vi "Test Process Restarting Maintains State.vi"(8 "error in (no error)":errorcluster, 11 "Process Test In":refnum<class "Process Test.lvclass">) -> (0 "error out":errorcluster, 3 "Process Test Out":refnum<class "Process Test.lvclass">)   [LabVIEW 2020, in "Process Test.lvclass"]
uses:
  Process Test.lvclass
  <vilib>/Asteme/LUnit/Test Case.lvclass
  C:/Program Files (x86)/National Instruments/LabVIEW 2020/vi.lib/Asteme/LUnit/Test Case.lvclass
  Framework/Process/Process.lvclass
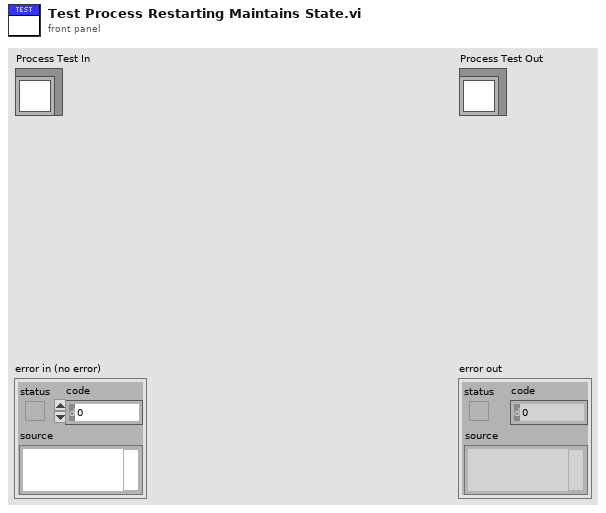
[diagram p1: front panel]
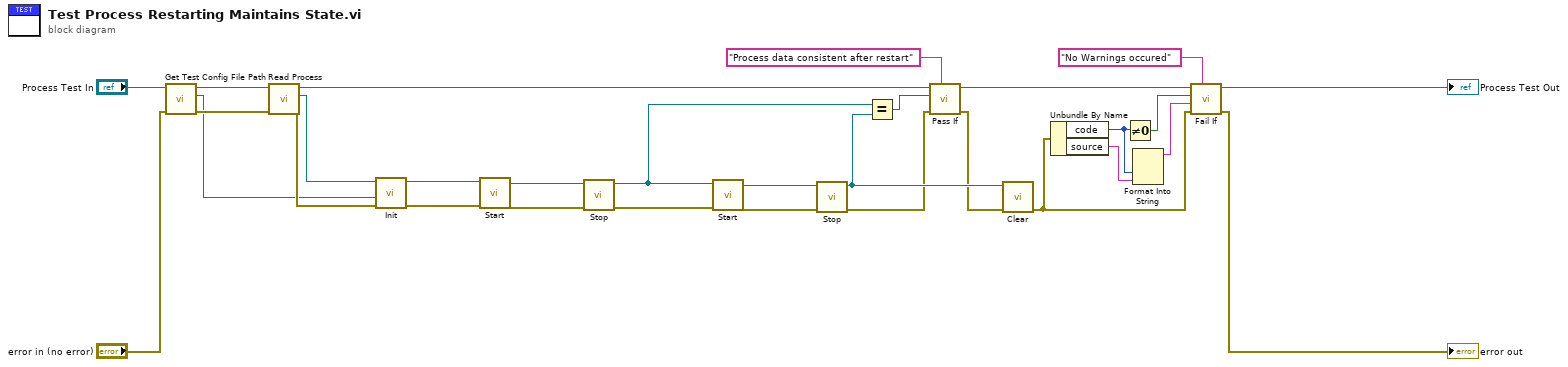
[diagram p0: block diagram]
diagram:
  n1 = call-dynamic "Get Test Config File Path.vi"("error in (no error)"="error in (no error)", "Base Class Test in"="Process Test In") -> ("error out"=w21:errorcluster, "Test config path"=w1:path, "Base Class Test out"=w25:refnum<class "Process Test.lvclass">)  [unwired: 7 in]
  n2 = call "Read Process.vi"("error in (no error)"=w21, "Process Test in"=w25) -> ("error out"=w22:errorcluster, "Process.lvclass"=w2:refnum<class "Process.lvclass">, "Process Test out"=w23:refnum<class "Process Test.lvclass">)  [unwired: 7 in]
  n3 = call-dynamic "Init.vi"("error in (no error)"=w22, "Config File Path"=w1, "Process In"=w2) -> ("error out"=w26:errorcluster, "Process Out"=w27:refnum<class "Process.lvclass">)  [unwired: 7 in]
  n4 = call "Start.vi"("error in (no error)"=w26, "Process In"=w27) -> ("error out"=w29:errorcluster, "Process Out"=w30:refnum<class "Process.lvclass">)  [unwired: 8 in]
  n5 = call "Stop.vi"("error in (no error)"=w29, "Process In"=w30) -> ("error out"=w3:errorcluster, "Process Out"=w10:refnum<class "Process.lvclass">)  [unwired: 7 in, 1 out]
  n6 = call "Start.vi"("error in (no error)"=w3, "Process In"=w10) -> ("error out"=w12:errorcluster, "Process Out"=w11:refnum<class "Process.lvclass">)  [unwired: 8 in]
  n7 = call "Stop.vi"("error in (no error)"=w12, "Process In"=w11) -> ("error out"=w6:errorcluster, "Process Out"=w9:refnum<class "Process.lvclass">)  [unwired: 7 in, 1 out]
  n8 = Equal?(x=w10, y=w9) -> (x = y?=w7:bool)
  n9 = call <vilib>:"Pass If.vi"("Description"="Process data consistent after restart", "error in (no error)"=w6, "Pass?"=w7, "Test Case In"=w23) -> ("error out"=w5:errorcluster, "Test Case Out"=w8:refnum<class "Process Test.lvclass">)  [unwired: 6 in]
  n10 = call-dynamic "Clear.vi"("error in (no error)"=w5, "Process In"=w9) -> ("error out"=w17:errorcluster)  [unwired: 9 in]
  n11 = Unbundle By Name(w17) -> ("code"=w15:i32, "source"=w13:string)
  n12 = Not Equal To 0?(x=w15) -> (x != 0?=w19:bool)
  n13 = Format Into String(w15, w13) -> (resulting string=w14:string)  [unwired: 3 in, 1 out]
  n14 = call <vilib>:"Fail If.vi"("Description"="No Warnings occured", "error in (no error)"=w17, "Message"=w14, "Fail?"=w19, "Test Case In"=w8) -> ("error out"=→"error out":errorcluster, "Test Case Out"=→"Process Test Out":refnum<class "Process Test.lvclass">)  [unwired: 5 in]
